vi "DSF.Engine.Framework.Get Plugin.vi"(10 "index":i32, 11 "Framework in":refnum<class "DSF.Engine.Framework.lvclass">) -> (2 "Plugin":refnum<class "DSF.Engine.Plugin.lvclass">, 3 "Framework out":refnum<class "DSF.Engine.Framework.lvclass">)   [LabVIEW 2017, in "DSF.Engine.lvlib" / "DSF.Engine.Framework.lvclass"]
uses:
  DSF.Engine.Framework.lvclass
  Plugin/DSF.Engine.Plugin.lvclass
  DSF.Engine.Framework.lvclass/DSF.Engine.Framework.ctl
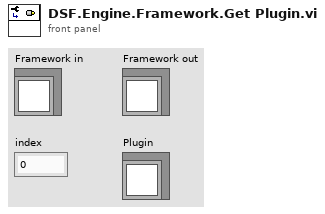
[diagram p1: front panel]
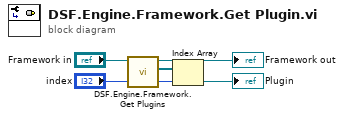
[diagram p0: block diagram]
diagram:
  n1 = call "DSF.Engine.Framework.Get Plugins.vi"("Framework in"="Framework in") -> ("Plugins"=w3:refnum<class "DSF.Engine.Plugin.lvclass">[], "Framework out"=→"Framework out":refnum<class "DSF.Engine.Framework.lvclass">)  [unwired: 9 in]
  n2 = Index Array(array=w3, index="index") -> (element=→"Plugin":refnum<class "DSF.Engine.Plugin.lvclass">)
